vi "OnDataChange.vi"(0 "GRMActor in":refnum<class "FlatFieldUI.lvclass">, 1 "DataExchange":T1, 3 "error in (no error)":errorcluster) -> (7 "GRMActor out":refnum<class "FlatFieldUI.lvclass">, 10 "error out":errorcluster)   [LabVIEW 2020, in "FlatFieldUI.lvlib" / "FlatFieldUI.lvclass"]
uses:
  FlatFieldUI.lvclass
  Hardware Abstraction Layer/Component/Device/Device/DataExchange.ctl
  FlatFieldUI.lvclass/FlatFieldUI.ctl
  Displayer/Displayer/FlatField Method.ctl
  FlatField/FlatField/FlatField Status.ctl
  Hardware Abstraction Layer/Component/GenericActor/GenericActor/GenericController.lvclass
  <vilib>/vision/NI_Vision_Development_Module.lvlib
  Interface/DataListener/DataListener.lvclass
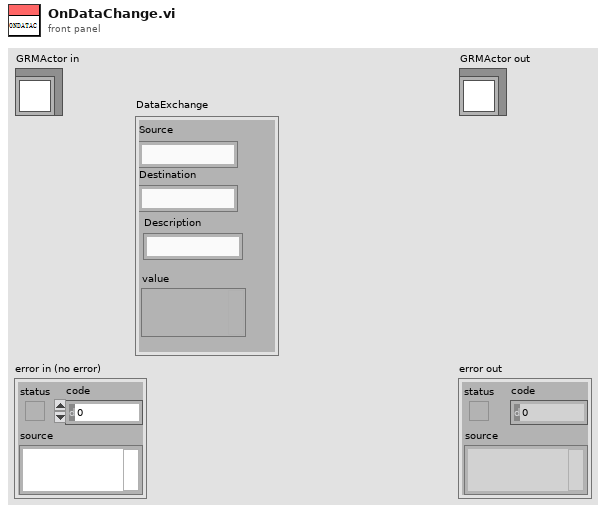
[diagram p1: front panel]
types:
  T1 = typedef "DataListener.lvclass/DataExchange.ctl" = cluster{"Source":string, "Destination":string, "Description":string, "value":variant}
  T2 = typedef "FlatFieldUI.lvlib/FlatFieldUI.lvclass/FlatField Method.ctl" = i32
  T3 = typedef "IMAQ Image.ctl" = refnum<image>
  T4 = typedef "FlatFieldUI.lvlib/FlatFieldUI.lvclass/FlatField Status.ctl" = i32
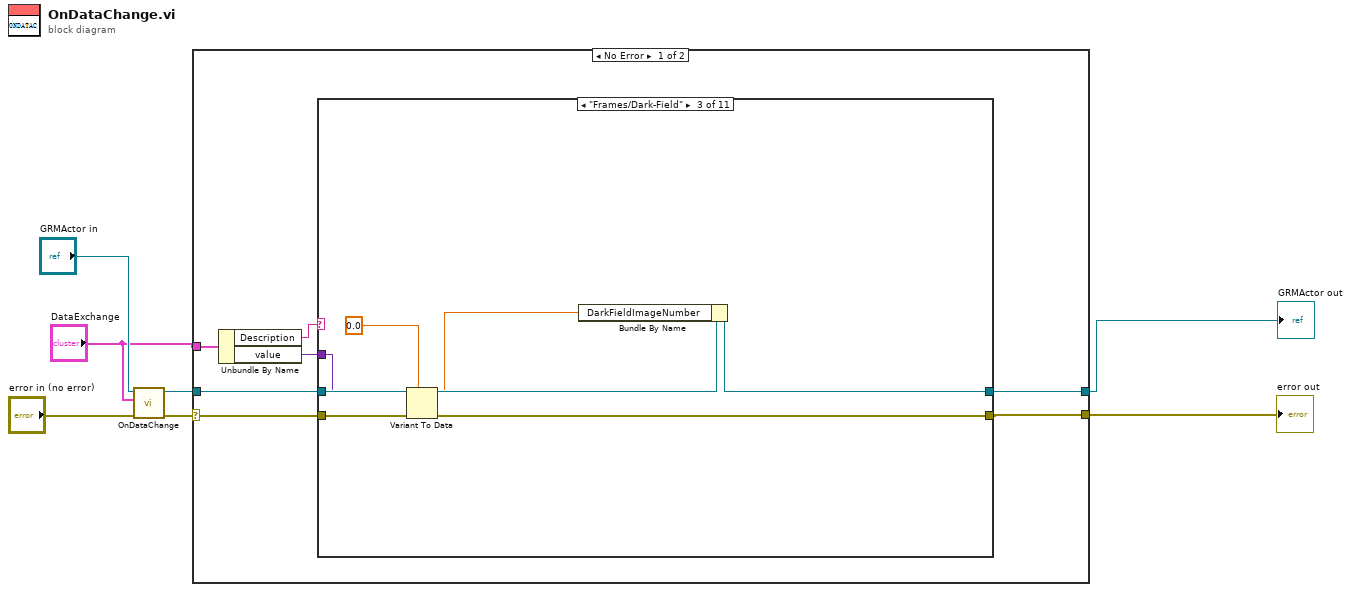
[diagram p0: block diagram]
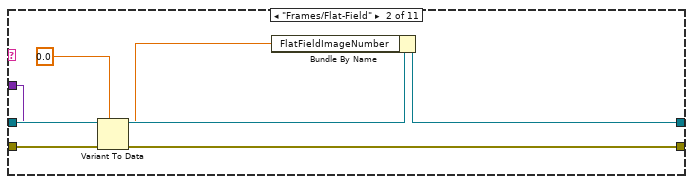
[diagram p3: hidden frame]
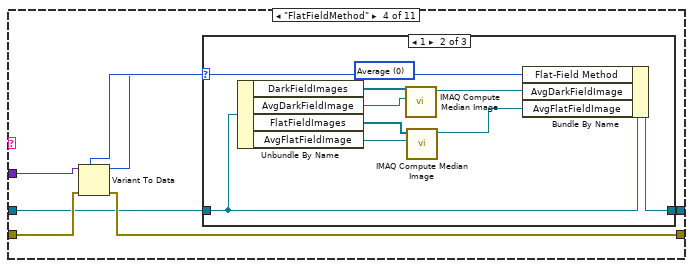
[diagram p4: hidden frame]
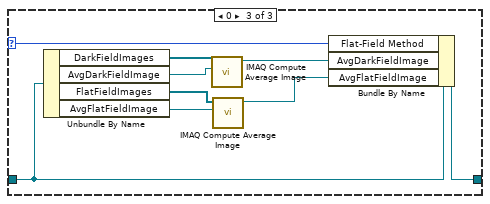
[diagram p6: hidden frame]
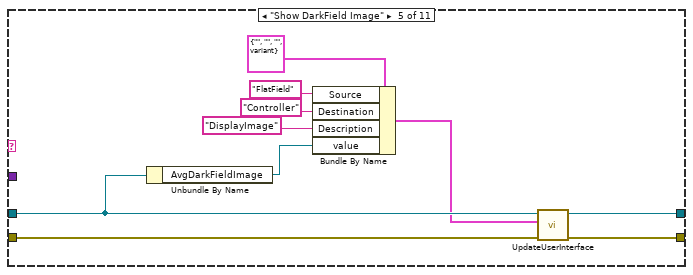
[diagram p7: hidden frame]
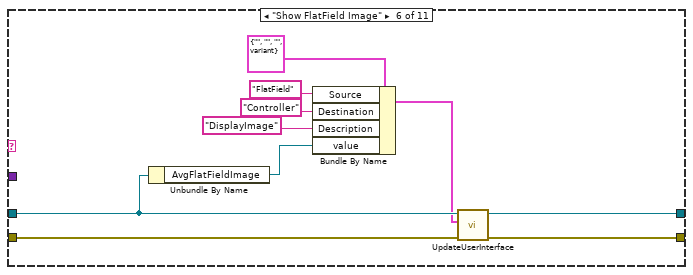
[diagram p8: hidden frame]
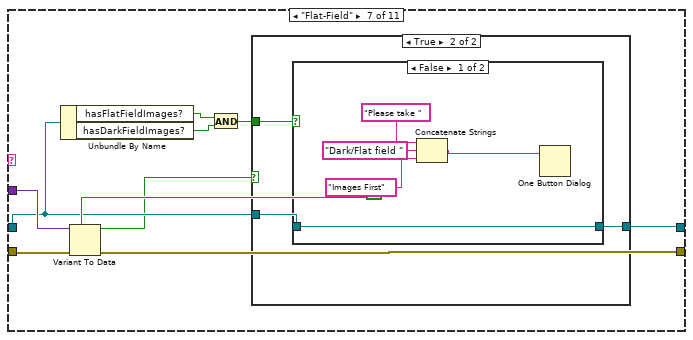
[diagram p9: hidden frame]
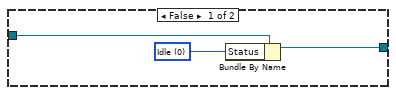
[diagram p10: hidden frame]
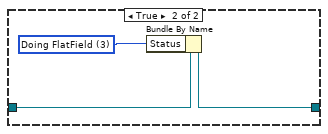
[diagram p11: hidden frame]
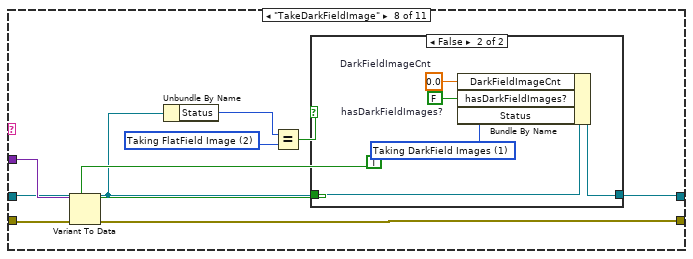
[diagram p12: hidden frame]
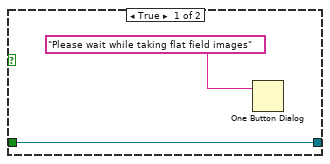
[diagram p13: hidden frame]
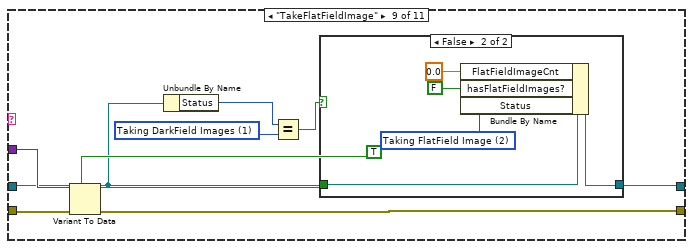
[diagram p14: hidden frame]
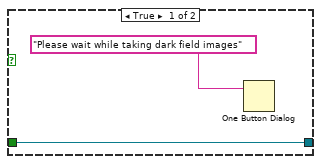
[diagram p15: hidden frame]
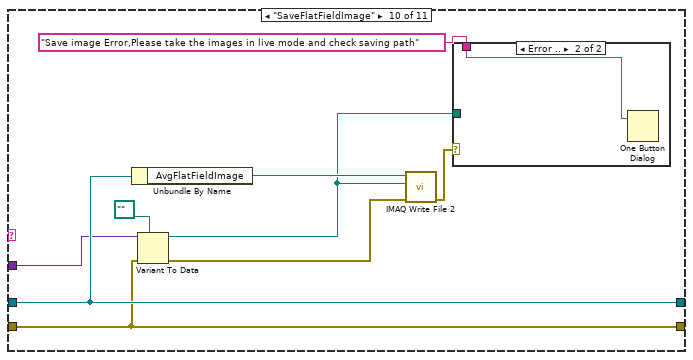
[diagram p16: hidden frame]
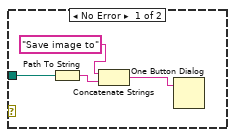
[diagram p17: hidden frame]
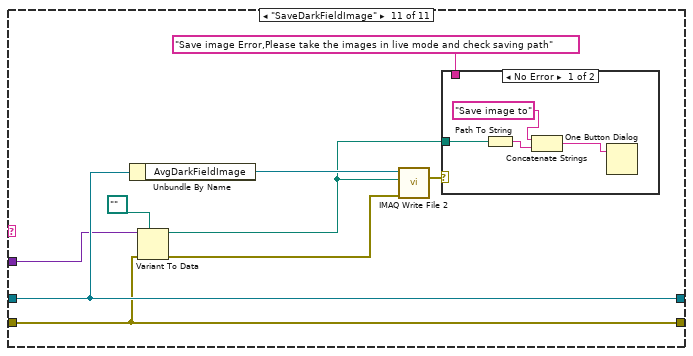
[diagram p18: hidden frame]
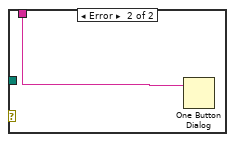
[diagram p19: hidden frame]
diagram:
  n1 = call-parent "OnDataChange.vi"("GRMActor in"="GRMActor in", "DataExchange"="DataExchange", "error in (no error)"="error in (no error)") -> ("GRMActor out"=w4:refnum<class "FlatFieldUI.lvclass">, "error out"=w5:errorcluster)  [unwired: 6 in]
  n2 = case shown="No Error" w5 {
    selector: w5 -> [w10 w163]
    tunnel: [w9 w163] -> w2
    tunnel: [w8 w164] -> w1
    tunnel: w4 -> [w11 w164]
    tunnel: "DataExchange" -> [w14 _]
    frame No Error {
      n3 = Unbundle By Name(w14) -> ("Description"=w13:string, "value"=w12:variant)
      n4 = case shown="\"Frames/Dark-Field\"" w13 {
        tunnel: w12 -> [_ w19 w26 w34 _ _ w84 w108 w125 w141 w155]
        tunnel: [w16 w21 w28 w33 w59 w69 w82 w106 w123 w143 w157] -> w8
        tunnel: w11 -> [w16 w23 w30 w32 w58 w68 w81 w104 w121 w143 w157]
        tunnel: [w15 w20 w27 w36 w60 w70 w85 w109 w126 w137 w151] -> w9
        tunnel: w10 -> [w15 w22 w29 w37 w61 w71 w86 w110 w127 w137 w151]
        frame Default {
        }
        frame "Frames/Flat-Field" {
          n5 = Variant To Data(error in=w22, type=0.0 ("FlatFieldImageNumber"), Variant=w19) -> (data=w17:dbl, error out=w20:errorcluster)
          n6 = Bundle By Name(cluster=w23, "FlatFieldImageNumber"=w17) -> (w21:refnum<class "FlatFieldUI.lvclass">)
        }
        frame "Frames/Dark-Field" {
          n7 = Variant To Data(error in=w29, type=0.0 ("FlatFieldImageNumber"), Variant=w26) -> (data=w24:dbl, error out=w27:errorcluster)
          n8 = Bundle By Name(cluster=w30, "DarkFieldImageNumber"=w24) -> (w28:refnum<class "FlatFieldUI.lvclass">)
        }
        frame "FlatFieldMethod" {
          w35 = T2 0 items=["Average", "Median"] ("Flat-Field Method")
          n9 = Variant To Data(error in=w37, type=w35, Variant=w34) -> (data=w31:T2, error out=w36:errorcluster)
          n10 = case shown="1" w31 {
            selector: w31 -> [_ w45 w54]
            tunnel: [w38 w47 w56] -> w33
            tunnel: w32 -> [w38 w46 w55]
            frame Default {
            }
            frame 1 {
              n11 = Unbundle By Name(w46) -> ("DarkFieldImages"=w44:T3[], "AvgDarkFieldImage"=w43:T3, "FlatFieldImages"=w41:T3[], "AvgFlatFieldImage"=w40:T3)
              n12 = call "IMAQ Compute Median Image"("Image Dst"=w43, "Images"=w44) -> ("Image Dst Out"=w42:T3)  [unwired: 8 in, 1 out]
              n13 = call "IMAQ Compute Median Image"("Image Dst"=w40, "Images"=w41) -> ("Image Dst Out"=w39:T3)  [unwired: 8 in, 1 out]
              n14 = Bundle By Name(cluster=w46, "Flat-Field Method"=w45, "AvgDarkFieldImage"=w42, "AvgFlatFieldImage"=w39) -> (w47:refnum<class "FlatFieldUI.lvclass">)
            }
            frame 0 {
              n15 = Unbundle By Name(w55) -> ("DarkFieldImages"=w53:T3[], "AvgDarkFieldImage"=w52:T3, "FlatFieldImages"=w50:T3[], "AvgFlatFieldImage"=w49:T3)
              n16 = call "IMAQ Compute Average Image"("Image Dst"=w52, "Images"=w53) -> ("Image Dst Out"=w51:T3)  [unwired: 8 in, 1 out]
              n17 = call "IMAQ Compute Average Image"("Image Dst"=w49, "Images"=w50) -> ("Image Dst Out"=w48:T3)  [unwired: 8 in, 1 out]
              n18 = Bundle By Name(cluster=w55, "Flat-Field Method"=w54, "AvgDarkFieldImage"=w51, "AvgFlatFieldImage"=w48) -> (w56:refnum<class "FlatFieldUI.lvclass">)
            }
          }
        }
        frame "Show DarkField Image" {
          n19 = Unbundle By Name(w58) -> ("AvgDarkFieldImage"=w62:T3)
          n20 = Bundle By Name(cluster=T1 {"Source"="", "Destination"="", "Description"="", "value"=variant} ("DataExchange"), "Source"="FlatField", "Destination"="Controller", "Description"="DisplayImage", "value"=w62) -> (w57:T1)
          n21 = call-dynamic "UpdateUserInterface.vi"("error in (no error)"=w61, "DataExchange"=w57, "FlatFieldUI in"=w58) -> ("error out"=w60:errorcluster, "FlatFieldUI out"=w59:refnum<class "FlatFieldUI.lvclass">)  [unwired: 6 in, 1 out]
        }
        frame "Show FlatField Image" {
          n22 = Unbundle By Name(w68) -> ("AvgFlatFieldImage"=w72:T3)
          n23 = Bundle By Name(cluster=T1 {"Source"="", "Destination"="", "Description"="", "value"=variant} ("DataExchange"), "Source"="FlatField", "Destination"="Controller", "Description"="DisplayImage", "value"=w72) -> (w67:T1)
          n24 = call-dynamic "UpdateUserInterface.vi"("error in (no error)"=w71, "DataExchange"=w67, "FlatFieldUI in"=w68) -> ("error out"=w70:errorcluster, "FlatFieldUI out"=w69:refnum<class "FlatFieldUI.lvclass">)  [unwired: 6 in, 1 out]
        }
        frame "Flat-Field" {
          n25 = Unbundle By Name(w81) -> ("hasFlatFieldImages?"=w80:bool, "hasDarkFieldImages?"=w79:bool)
          n26 = Variant To Data(error in=w86, type=TRUE ("Boolean"), Variant=w84) -> (data=w77:bool, error out=w85:errorcluster)
          n27 = And(x=w80, y=w79) -> (x .and. y?=w78:bool)
          n28 = case shown="True" w77 {
            tunnel: [w88 w92] -> w82
            tunnel: w81 -> [w89 w91]
            tunnel: w78 -> [_ w90]
            frame False {
              w87 = T4 0 items=["Idle", "Taking DarkField Images", "Taking FlatField Image", "Doing FlatField", ""] ("Flat-Field Status")
              n29 = Bundle By Name(cluster=w89, "Status"=w87) -> (w88:refnum<class "FlatFieldUI.lvclass">)
            }
            frame True {
              n30 = case shown="False" w90 {
                tunnel: w91 -> [w93 w100]
                tunnel: [w93 w99] -> w92
                frame False {
                  n31 = Concatenate Strings("Please take " ("message"), "Dark/Flat field " ("string"), "Images First" ("string")) -> (w96:string)
                  n32 = One Button Dialog(message=w96) -> ()  [unwired: 1 in, 1 out]
                }
                frame True {
                  w98 = T4 3 items=["Idle", "Taking DarkField Images", "Taking FlatField Image", "Doing FlatField", ""] ("Flat-Field Status")
                  n33 = Bundle By Name(cluster=w100, "Status"=w98) -> (w99:refnum<class "FlatFieldUI.lvclass">)
                }
              }
            }
          }
        }
        frame "TakeDarkFieldImage" {
          w102 = T4 2 items=["Idle", "Taking DarkField Images", "Taking FlatField Image", "Doing FlatField", ""] ("y")
          n34 = Variant To Data(error in=w110, type=TRUE ("Boolean"), Variant=w108) -> (data=w105:bool, error out=w109:errorcluster)
          n35 = Unbundle By Name(w104) -> ("Status"=w103:T4)
          n36 = Equal?(x=w103, y=w102) -> (x = y?=w101:bool)
          n37 = case shown="False" w101 {
            tunnel: w104 -> [w112 w113]
            tunnel: [w112 w117] -> w106
            tunnel: w105 -> [_ _]
            frame True {
              n38 = One Button Dialog(message="Please wait while taking flat field images") -> ()  [unwired: 1 in, 1 out]
            }
            frame False {
              w114 = T4 1 items=["Idle", "Taking DarkField Images", "Taking FlatField Image", "Doing FlatField", ""] ("Flat-Field Status")
              w115 = 0.0  # DarkFieldImageCnt
              w116 = FALSE  # hasDarkFieldImages?
              n39 = Bundle By Name(cluster=w113, "DarkFieldImageCnt"=w115, "hasDarkFieldImages?"=w116, "Status"=w114) -> (w117:refnum<class "FlatFieldUI.lvclass">)
            }
          }
        }
        frame "TakeFlatFieldImage" {
          w119 = T4 1 items=["Idle", "Taking DarkField Images", "Taking FlatField Image", "Doing FlatField", ""] ("y")
          n40 = Variant To Data(error in=w127, type=TRUE ("Boolean"), Variant=w125) -> (data=w122:bool, error out=w126:errorcluster)
          n41 = Unbundle By Name(w121) -> ("Status"=w120:T4)
          n42 = Equal?(x=w120, y=w119) -> (x = y?=w118:bool)
          n43 = case shown="False" w118 {
            tunnel: w121 -> [w129 w130]
            tunnel: [w129 w134] -> w123
            tunnel: w122 -> [_ _]
            frame True {
              n44 = One Button Dialog(message="Please wait while taking dark field images") -> ()  [unwired: 1 in, 1 out]
            }
            frame False {
              w131 = T4 2 items=["Idle", "Taking DarkField Images", "Taking FlatField Image", "Doing FlatField", ""] ("Flat-Field Status")
              n45 = Bundle By Name(cluster=w130, "FlatFieldImageCnt"=0.0 ("DarkFieldImageCnt"), "hasFlatFieldImages?"=FALSE ("hasDarkFieldImages?"), "Status"=w131) -> (w134:refnum<class "FlatFieldUI.lvclass">)
            }
          }
        }
        frame "SaveFlatFieldImage" {
          n46 = Unbundle By Name(w143) -> ("AvgFlatFieldImage"=w142:T3)
          n47 = Variant To Data(error in=w137, type=path "" ("Path"), Variant=w141) -> (data=w138:path, error out=w139:errorcluster)
          n48 = call-poly "IMAQ Write File 2"("error in (no error)"=w139, "File Path"=w138, "Image"=w142) -> ("error out"=w136:errorcluster)  [unwired: 7 in, 1 out]
          n49 = case shown="Error .." w136 {
            tunnel: w138 -> [w147 _]
            tunnel: "Save image Error,Please take the images in live mode and check saving path" ("message") -> [_ w148]
            frame No Error {
              n50 = Path To String(path=w147) -> (string=w145:string)
              n51 = Concatenate Strings("Save image to" ("message"), w145) -> (w144:string)
              n52 = One Button Dialog(message=w144) -> ()  [unwired: 1 in, 1 out]
            }
            frame Error {
              n53 = One Button Dialog(message=w148) -> ()  [unwired: 1 in, 1 out]
            }
          }
        }
        frame "SaveDarkFieldImage" {
          n54 = Unbundle By Name(w157) -> ("AvgDarkFieldImage"=w156:T3)
          n55 = Variant To Data(error in=w151, type=path "" ("Path"), Variant=w155) -> (data=w152:path, error out=w153:errorcluster)
          n56 = call-poly "IMAQ Write File 2"("error in (no error)"=w153, "File Path"=w152, "Image"=w156) -> ("error out"=w150:errorcluster)  [unwired: 7 in, 1 out]
          n57 = case shown="No Error" w150 {
            tunnel: w152 -> [w161 _]
            tunnel: "Save image Error,Please take the images in live mode and check saving path" ("message") -> [_ w162]
            frame No Error {
              n58 = Path To String(path=w161) -> (string=w159:string)
              n59 = Concatenate Strings("Save image to" ("message"), w159) -> (w158:string)
              n60 = One Button Dialog(message=w158) -> ()  [unwired: 1 in, 1 out]
            }
            frame Error {
              n61 = One Button Dialog(message=w162) -> ()  [unwired: 1 in, 1 out]
            }
          }
        }
      }
    }
    frame Error {
    }
  }
  "error out" <- w2
  "GRMActor out" <- w1
